vi "Find Point Correspondences.vi"(7 "Point Correspondence Params (Default: pcl Defaults) in":refnum<class "Point Correspondence Params.lvclass">, 8 "error in (no error)":errorcluster, 10 "Target Points":T2[](array[typedef]), 11 "Source Points":T2[](array[typedef])) -> (0 "error out":errorcluster, 3 "Correspondences":T1[](array[typedef]))   [LabVIEW 2020, in "ar.lvlib"]
doc: "Find the correspondences between two unordered 3D Point Sets. This uses the PCL (point cloud library) function pcl::registration::CorrespondenceRejectorSampleConsensus. More details can be found at https://pointclouds.org/documentation/classpcl_1_1registration_1_1_correspondence_rejector_sample_consensus.html"
uses:
  ar.lvlib
  common/Object Point (Float).ctl
  Correspondence Index.ctl
  Point Correspondence Params/Point Correspondence Params.lvclass
  Point Correspondence Params/Point Correspondence Params.lvclass/Point Correspondence Params.ctl
  common/common.lvlib
  common/bin/gartoolkit_32-1.dll
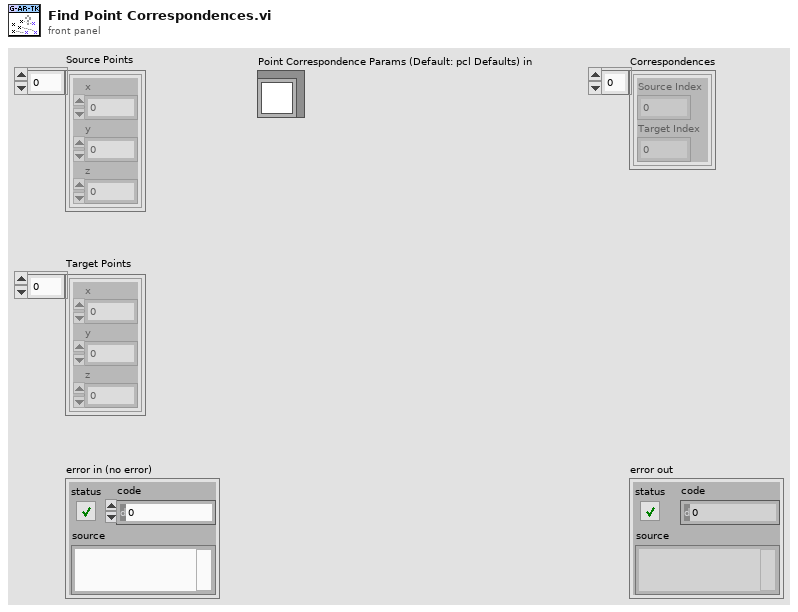
[diagram p1: front panel]
types:
  T1 = typedef "ar.lvlib/Correspondence Index.ctl" = cluster{"Source Index":i32, "Target Index":i32}
  T2 = typedef "common.lvlib/Object Point (Float).ctl" = cluster{"x":dbl, "y":dbl, "z":dbl}
  T3 = typedef "ar.lvlib/Point Correspondence Params.lvclass/Params.ctl" = cluster{"Refine":bool, "Max Iterations":i32, "Inlier Threshold":dbl}
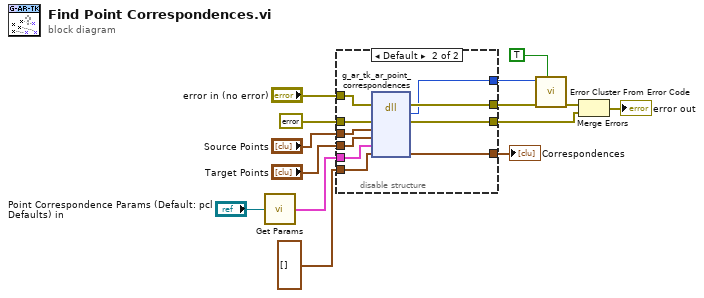
[diagram p0: block diagram]
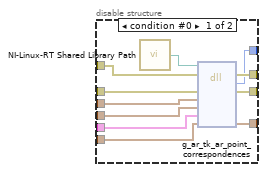
[diagram p2: hidden frame]
diagram:
  n1 = call "Get Params.vi"("Point Correspondence Params in"="Point Correspondence Params (Default: pcl Defaults) in") -> ("Params"=w2:T3)
  n2 = disable-structure shown="Default" {
    disable-tunnel: "error in (no error)" -> [w24 w35]
    disable-tunnel: errorcluster {"status"=FALSE, "code"=0, "source"=""} ("error constant") -> [w23 w31]
    disable-tunnel: [w22 w34] -> w14
    disable-tunnel: [w21 w33] -> w13
    disable-tunnel: [w20 w32] -> w12
    disable-tunnel: "Source Points" -> [w19 w30]
    disable-tunnel: "Target Points" -> [w18 w29]
    disable-tunnel: w2 -> [w17 w28]
    disable-tunnel: T1[] [] -> [w16 w27]
    disable-tunnel: [w15 w26] -> w4
    frame condition #0 {
      n3 = call "NI-Linux-RT Shared Library Path.vi"() -> ("Path"=w25:path)
      n4 = dll-call lib="?" fn="g_ar_tk_ar_point_correspondences" ("g_ar_toolkit.*.*:g_ar_tk_image_copy")(path in=w25, error in=w24, "error_cluster"=w23, "source_points"=w19, "target_points"=w18, "params"=w17, "correspondences"=w16) -> (error out=w22:errorcluster, "MgErr"=w21:i32, "error_cluster"=w20:errorcluster, "correspondences"=w15:T1[])  [unwired: 4 in, 1 out]
    }
    frame condition #1 (active) {
      n5 = dll-call lib="C:/serenial/lib/g-augmented-reality-toolkit/LabVIEW/common/bin/gartoolkit_*-1.*" fn="g_ar_tk_ar_point_correspondences" ("g_ar_toolkit.*.*:g_ar_tk_image_copy")(error in=w35, "error_cluster"=w31, "source_points"=w30, "target_points"=w29, "params"=w28, "correspondences"=w27) -> (error out=w34:errorcluster, "MgErr"=w33:i32, "error_cluster"=w32:errorcluster, "correspondences"=w26:T1[])  [unwired: 5 in, 1 out]
    }
  }
  "Correspondences" <- w4
  n6 = call <vilib>:"Error Cluster From Error Code.vi"("show call chain? (False)"=TRUE, "error in (no error)"=w14, "error code (0)"=w13) -> ("error out"=w11:errorcluster)  [unwired: 6 in]
  n7 = Merge Errors(w11, w12) -> (→"error out":errorcluster)
